vi "App Main.vi"(11 "Ready Notifier":refnum<notifier>) -> ()   [LabVIEW 2020, in "PicoG-App.lvlib"]
uses:
  PicoG-App.lvlib
  App/App.lvclass
types:
  T1 = enum32{"invalid app kind", "Development System", "Run Time System", "Student Edition", "Embedded LabVIEW", "Evaluation", "Custom"}
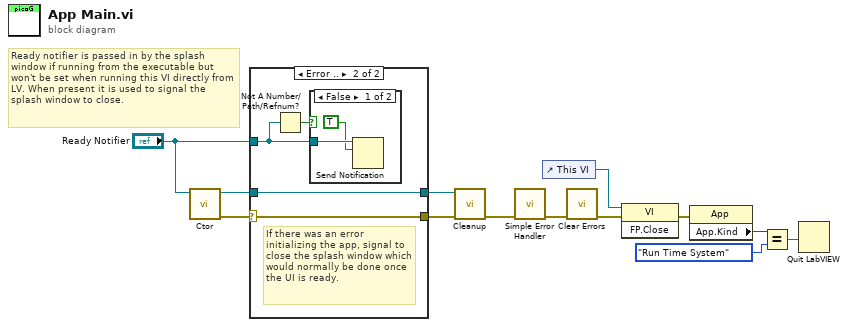
[diagram p0: block diagram]
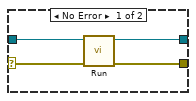
[diagram p2: hidden frame]
diagram:
  # "Ready notifier is passed in by the splash window if running from the executable but won't be set when running this VI directly from LV. When present it is used to signal the splash window to close."
  n1 = call "Ctor.vi"("Ready Notifier"="Ready Notifier") -> ("error out"=w8:errorcluster, "App out"=w7:refnum<class "App.lvclass">)  [unwired: 9 in]
  n2 = case shown="Error .." w8 {
    selector: w8 -> [w16 w18]
    tunnel: "Ready Notifier" -> [_ w20]
    tunnel: w7 -> [w17 w19]
    tunnel: [w15 w18] -> w5
    tunnel: [w14 w19] -> w6
    frame No Error {
      n3 = call "Run.vi"("error in (no error)"=w16, "App in"=w17) -> ("error out"=w15:errorcluster, "App out"=w14:refnum<class "App.lvclass">)  [unwired: 8 in]
    }
    frame Error {
      # "If there was an error initializing the app, signal to close the splash window which would normally be done once the UI is ready."
      n4 = Not A Number/Path/Refnum?(number/path/refnum=w20) -> (NaN/Path/Refnum?=w21:bool)
      n5 = case shown="False" w21 {
        tunnel: w20 -> [w23 _]
        frame False {
          n6 = Send Notification(notification=TRUE, notifier=w23) -> ()  [unwired: 1 in, 2 out]
        }
        frame True {
        }
      }
    }
  }
  n7 = call "Cleanup.vi"("error in (no error)"=w5, "App in"=w6) -> ("error out"=w3:errorcluster)  [unwired: 9 in]
  n8 = call <vilib>:"Simple Error Handler.vi"("error in (no error)"=w3) -> ("error out"=w2:errorcluster)  [unwired: 4 in, 4 out]
  n9 = control-ref of="This VI"() -> (w4:refnum<vi>)
  n10 = call <vilib>:"Clear Errors.vi"("error in (no error)"=w2) -> ("error out"=w1:errorcluster)  [unwired: 5 in, 1 out]
  n11 = invoke class="VI" method="FP.Close"(reference=w4, error in=w1) -> (error out=w10:errorcluster)  [unwired: 1 in, 2 out]
  n12 = property class="App"(error in=w10) -> ("App.Kind"=w13:T1)  [unwired: 1 in, 2 out]
  n13 = Equal?(x=w13, y=T1."Run Time System" ("Application:Kind")) -> (x = y?=w11:bool)
  n14 = Quit LabVIEW(quit? (T)=w11) -> ()
